vi "TLTSP_Measurement.vi"(8 "error in (no error)":errorcluster, 10 "Select Measurement":i32(ring) items=["Temperature", "Humidity", "TH1", "TH2"], 11 "VISA resource name":refnum<visa-resource-name>) -> (0 "error out":errorcluster, 2 "Output":string, 3 "VISA resource name out":refnum<visa-resource-name>)   [LabVIEW 2017]
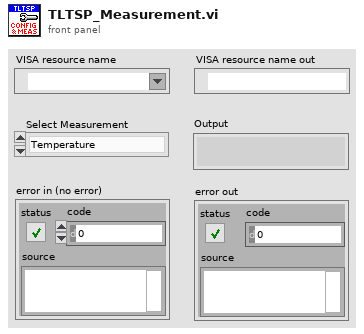
[diagram p1: front panel]
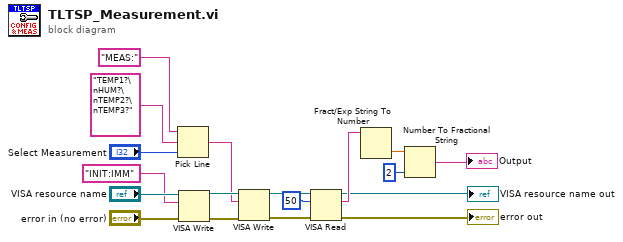
[diagram p0: block diagram]
diagram:
  n1 = Pick Line(string ("")="MEAS:", multi-line string="TEMP1?\nHUM?\nTEMP2?\nTEMP3?", line index="Select Measurement") -> (output string=w3:string)
  n2 = VISA Write(VISA resource name="VISA resource name", write buffer="INIT:IMM", error in (no error)="error in (no error)") -> (VISA resource name out=w8:refnum<visa-resource-name>, error out=w11:errorcluster)  [unwired: 1 out]
  n3 = VISA Write(VISA resource name=w8, write buffer=w3, error in (no error)=w11) -> (VISA resource name out=w9:refnum<visa-resource-name>, error out=w10:errorcluster)  [unwired: 1 out]
  n4 = VISA Read(VISA resource name=w9, byte count=u32 50, error in (no error)=w10) -> (VISA resource name out=→"VISA resource name out":refnum<visa-resource-name>, read buffer=w12:string, error out=→"error out":errorcluster)  [unwired: 1 out]
  n5 = Fract/Exp String To Number(string=w12) -> (number=w14:dbl)  [unwired: 3 in, 1 out]
  n6 = Number To Fractional String(number=w14, precision (6)=i16 2) -> (F-format string=→"Output":string)  [unwired: 2 in]
